vi "user_agent.vi"() -> (3 "header":cluster{"header":string, "value":string}={"header"="Content-Type", "value"="application/json"})   [LabVIEW 2015, in "lv-dropbox.lvlib"]
uses:
  lv-dropbox.lvlib
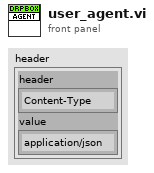
[diagram p1: front panel]
types:
  T1 = typedef "lv-dropbox.lvlib/content_type.ctl" = enum16{"<content_type>", "json"}
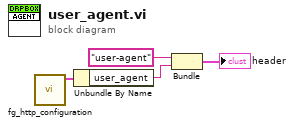
[diagram p0: block diagram]
diagram:
  n1 = call "fg_http_configuration.vi"() -> ("http_configuration out"=w3:cluster{"content_type":T1, "user_agent":string})  [unwired: 10 in, 1 out]
  n2 = Unbundle By Name(w3) -> ("user_agent"=w2:string)
  n3 = Bundle("header"="user-agent", "user_agent"=w2) -> (→"header":cluster{"header":string, "user_agent":string})  [unwired: 1 in]
